vi "Kill Loader.vi"(10 "Log":bool=TRUE, 11 "PIDs":u32[](array[numeric])) -> (0 "error out":errorcluster, 2 "Failed to stop":bool, 3 "Kill Action":T1(ring))   [LabVIEW 2021, in "CIFPluginManager.lvclass"]
uses:
  CIFPluginManager.lvclass
  <vilib>/CIF Foundation/CIF Core/CIFCore/Common/Typedef/Errors.ctl
  typedef/Kill Statemachine.ctl
  <vilib>/CIF Foundation/CIF Core/CIFUtilities/CIFLogs/Typedef/Message Type.ctl
  <vilib>/CIF Foundation/CIF Utilities/Errors/Append Error Location.vi
  <vilib>/CIF Foundation/CIF Core/CIFUtilities/CIFLogs/CIFLogs.lvlib
  <vilib>/CIF Foundation/CIF Core/CIFCore/Common/CIFCoreCommon.lvlib
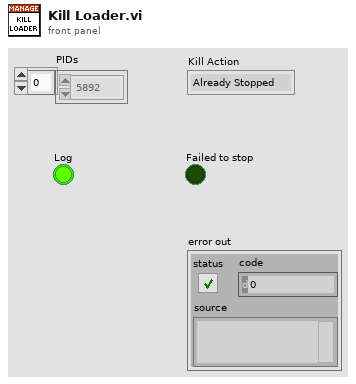
[diagram p1: front panel]
types:
  T1 = enum16{"Already Stopped", "SigInt", "SigTerm", "SigKill"}
  T2 = typedef "CIFCoreCommon.lvlib/Errors.ctl" = enum16{"Invalid Clock ID", "Long Sleep", "gRPC Server Not Found", "Config Parse", "Timestamp Wrap", "Delayed Execution", "Duplicate Channel", "Missing Channel", "Incorrect Type", "Flatten Error", "Unflatten Data", "Unique Name", "Plugin Not Found", "Plugin Type Not Found", "Plugin Version Not Found", "Manager Not Found", "Numerical Issue", "Time Jump", "Clock ID Match", "Channel Length", "Plugin Connection", "gRPC Server Connection", "PPL Name Match", "Build", "Config Log Parse", "Plugin Load", "UI Subpanel Load", "Python Name", "Invalid Name", "Unable to Change Ch Buffer", "Failed Kill", "Failed SysExec", "Function Not Implemented", "Load Timeout"}
  T3 = typedef "CIFPluginManager.lvclass/Kill Statemachine.ctl" = enum16{"Check for Running", "Sleep", "SigInt", "SigTerm", "SigKill"}
  T4 = typedef "CIFLogs.lvlib/Message Type.ctl" = enum16{"Error", "Information", "Print Terminal", "Configuration"}
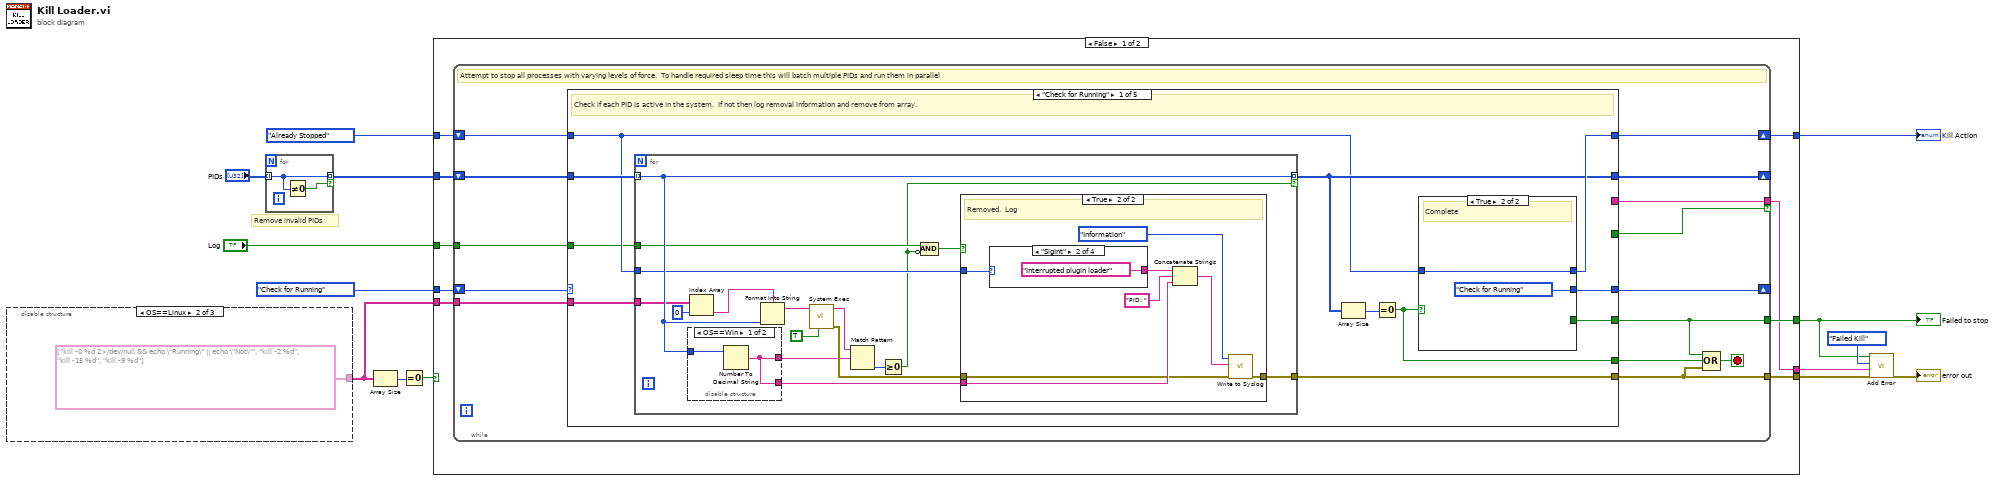
[diagram p0: block diagram]
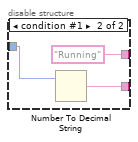
[diagram p2: hidden frame]
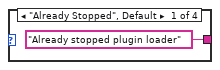
[diagram p4: hidden frame]
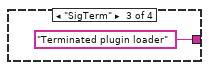
[diagram p5: hidden frame]
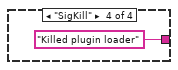
[diagram p6: hidden frame]
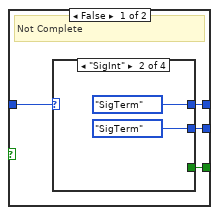
[diagram p7: hidden frame]
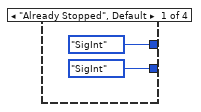
[diagram p8: hidden frame]
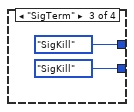
[diagram p9: hidden frame]
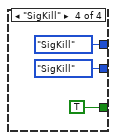
[diagram p10: hidden frame]
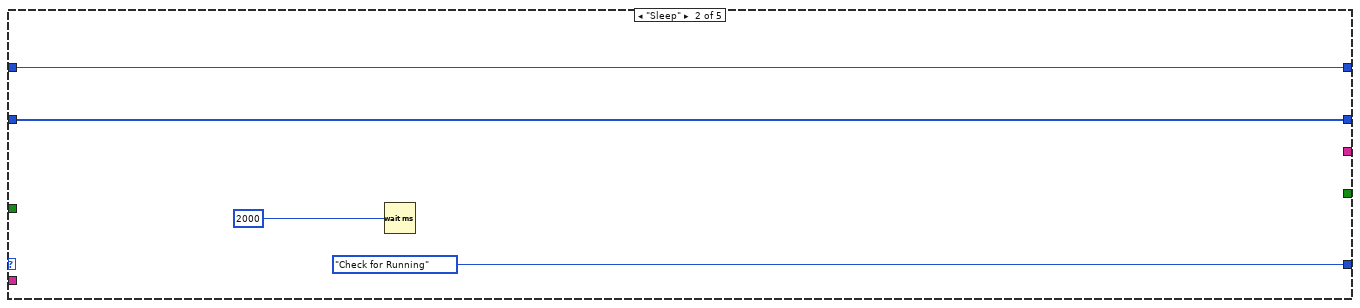
[diagram p11: hidden frame]
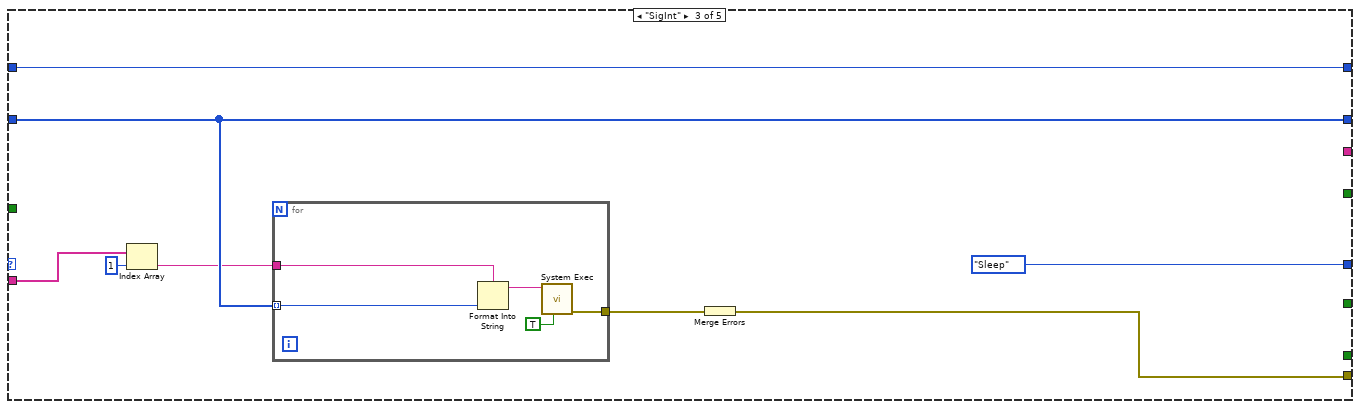
[diagram p12: hidden frame]
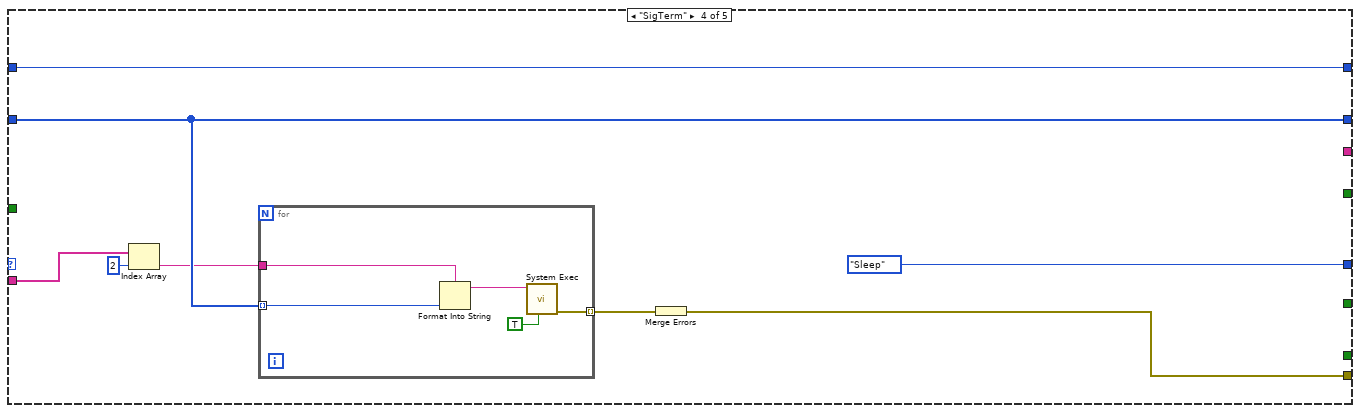
[diagram p13: hidden frame]
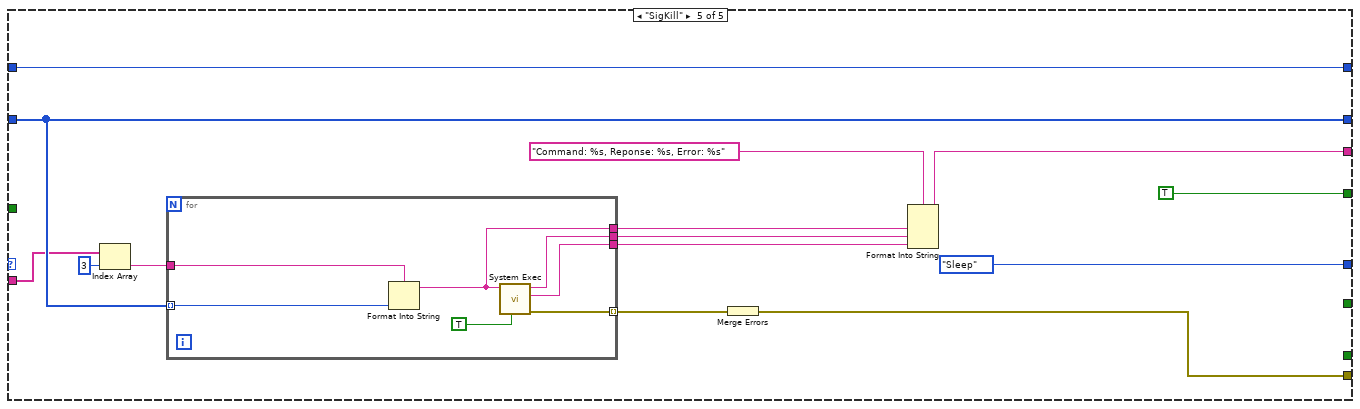
[diagram p14: hidden frame]
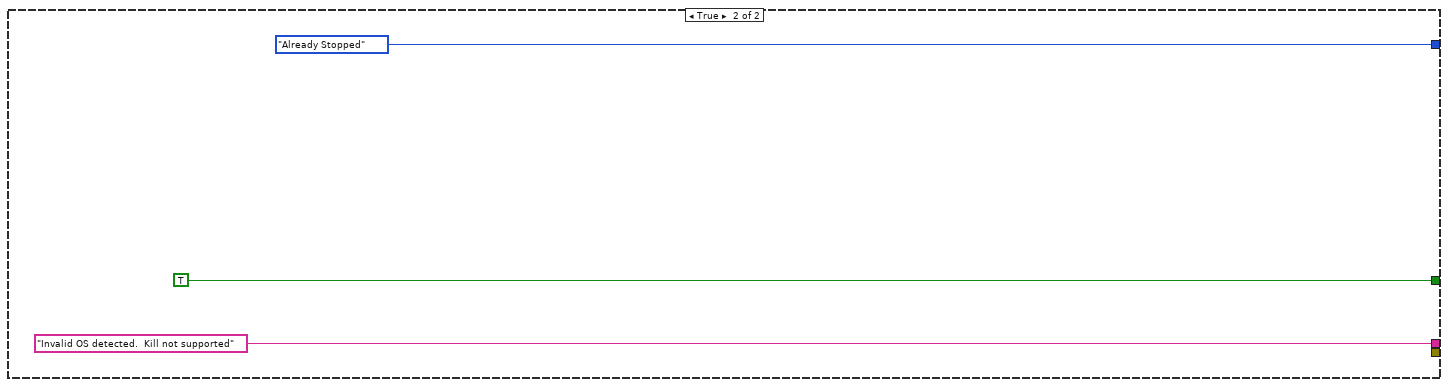
[diagram p15: hidden frame]
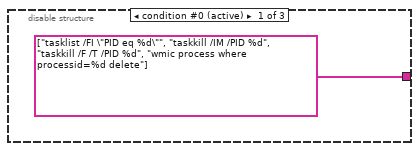
[diagram p16: hidden frame]
diagram:
  # "Remove invalid PIDs"
  n1 = disable-structure shown="OS==Linux" {
    disable-tunnel: [string[] ["tasklist /FI \"PID eq %d\"", "taskkill /IM /PID %d", "taskkill /F /T /PID %d", "wmic process where processid=%d delete"] string[] ["kill -0 %d 2>/dev/null && echo \"Running\" || echo \"Not\"", "kill -2 %d", "kill -15 %d", "kill -9 %d"] _] -> w3
    frame condition #0 (active) {
    }
    frame condition #1 {
    }
    frame condition #2 {
    }
  }
  n2 = for {
    tunnel: "PIDs" -> [w18] mode=indexing
    tunnel: [w18] -> w10 mode=indexing if=w17
    n3 = Not Equal To 0?(x=w18) -> (x != 0?=w17:bool)
  }
  n4 = Array Size(array=w3) -> (size(s)=w4:i32)
  n5 = Equal To 0?(x=w4) -> (x = 0?=w1:bool)
  n6 = case shown="False" w1 {
    tunnel: Kill_Statemachine."Check for Running" ("Kill Statemachine") -> [w27 _]
    tunnel: T1."Already Stopped" ("Kill Result") -> [w26 _]
    tunnel: [w25 T1."Already Stopped" ("Kill Result")] -> w12
    tunnel: w10 -> [w24 _]
    tunnel: [w23 _] -> w8
    tunnel: [w22 TRUE] -> w2
    tunnel: [w21 "Invalid OS detected.  Kill not supported"] -> w6
    tunnel: "Log" -> [w20 _]
    tunnel: w3 -> [w19 _]
    frame False {
      n7 = while {
        shift-right: [w39] -> _
        shift-left: w27 -> [w41]
        shift-right: [w38] -> w25
        shift-left: w26 -> [w40]
        tunnel: [w31] -> w22
        tunnel: [w36] -> w21 if=w35
        tunnel: [w34] -> w23
        shift-right: [w32] -> _
        shift-left: w24 -> [w33]
        tunnel: w20 -> [w29]
        tunnel: w19 -> [w28]
        stop <- w37 stop-if-true
        # "Attempt to stop all processes with varying levels of force.  To handle required sleep time this will batch multiple PIDs and run them in parallel"
        n8 = case shown="\"Check for Running\"" w41 {
          tunnel: [w45 _ _ _ _] -> w30
          tunnel: w40 -> [w44 w105 w113 w126 w145]
          tunnel: [w52 w105 w113 w126 w145] -> w38
          tunnel: [w51 Kill_Statemachine."Check for Running" ("Kill Statemachine") Kill_Statemachine."Sleep" ("Kill Statemachine") Kill_Statemachine."Sleep" ("Kill Statemachine") Kill_Statemachine."Sleep" ("Kill Statemachine")] -> w39
          tunnel: [w50 _ _ _ _] -> w31
          tunnel: [_ _ _ _ w139] -> w36
          tunnel: [_ _ _ _ TRUE] -> w35
          tunnel: [w49 _ w109 w123 w136] -> w34
          tunnel: w33 -> [w48 w102 w111 w122 w135]
          tunnel: [w46 w102 w111 w122 w135] -> w32
          tunnel: w29 -> [w43 _ _ _ _]
          tunnel: w28 -> [w42 _ w107 w119 w132]
          frame "Check for Running" {
            # "Check if each PID is active in the system.  If not then log removal information and remove from array."
            n9 = for {
              tunnel: [w61] -> w49
              tunnel: w48 -> [w64] mode=indexing
              tunnel: [w64] -> w46 mode=indexing if=w59
              tunnel: w44 -> [w63]
              tunnel: w43 -> [w60]
              tunnel: w42 -> [w57]
              n10 = disable-structure shown="OS==Win" {
                disable-tunnel: w64 -> [w70 w72]
                disable-tunnel: [w69 "Running"] -> w54
                disable-tunnel: [w69 w71] -> w53
                frame condition #0 (active) {
                  n11 = Number To Decimal String(number=w70) -> (decimal integer string=w69:string)  [unwired: 1 in]
                }
                frame condition #1 {
                  n12 = Number To Decimal String(number=w72) -> (decimal integer string=w71:string)  [unwired: 1 in]
                }
              }
              n13 = Index Array(array=w57, index=0) -> (element=w56:string)
              n14 = Format Into String(format string=w56, w64) -> (resulting string=w68:string)  [unwired: 2 in, 1 out]
              n15 = call <vilib>:"System Exec.vi"("run minimized? (F)"=TRUE, "command line"=w68) -> ("error out"=w62:errorcluster, "standard output"=w66:string)  [unwired: 6 in, 2 out]
              n16 = Match Pattern(string=w66, regular expression=w54) -> (offset past match=w65:i32)  [unwired: 1 in, 3 out]
              n17 = Greater Or Equal To 0?(x=w65) -> (x >= 0?=w59:bool)
              n18 = Compound Arithmetic op=AND(w60, invert w59) -> (w58:bool)
              n19 = case shown="True" w58 {
                tunnel: w53 -> [_ w81]
                tunnel: w63 -> [_ w79]
                tunnel: w62 -> [w74 w77]
                tunnel: [w74 w76] -> w61
                frame False {
                  # "Not Removed"
                }
                frame True {
                  # "Removed.  Log"
                  n20 = case shown="\"SigInt\"" w79 {
                    tunnel: ["Already stopped plugin loader" ("message") "Interrupted plugin loader" ("message") "Terminated plugin loader" ("message") "Killed plugin loader" ("message")] -> w82
                    frame "Already Stopped", Default {
                    }
                    frame "SigInt" {
                    }
                    frame "SigTerm" {
                    }
                    frame "SigKill" {
                    }
                  }
                  n21 = Concatenate Strings(w82, "PID: " ("message"), w81) -> (w75:string)
                  n22 = call <vilib>:"Write to Syslog.vi"("error in (no error)"=w77, "message"=w75, "CIF Message Type"=Message_Type."Information") -> ("error out"=w76:errorcluster)  [unwired: 8 in]
                }
              }
            }
            n23 = Array Size(array=w46) -> (size(s)=w47:i32)
            n24 = Equal To 0?(x=w47) -> (x = 0?=w45:bool)
            n25 = case shown="True" w45 {
              tunnel: w44 -> [w90 w101]
              tunnel: [w88 w101] -> w52
              tunnel: [w89 Kill_Statemachine."Check for Running" ("Kill Statemachine")] -> w51
              tunnel: [w87 _] -> w50
              frame False {
                # "Not Complete"
                n26 = case shown="\"SigInt\"" w90 {
                  tunnel: [Kill_Statemachine."SigInt" ("Kill Statemachine") Kill_Statemachine."SigTerm" ("Kill Statemachine") Kill_Statemachine."SigKill" ("Kill Statemachine") Kill_Statemachine."SigKill" ("Kill Statemachine")] -> w89
                  tunnel: [T1."SigInt" ("Kill Result") T1."SigTerm" ("Kill Result") T1."SigKill" ("Kill Result") T1."SigKill" ("Kill Result")] -> w88
                  tunnel: [_ _ _ TRUE] -> w87
                  frame "Already Stopped", Default {
                  }
                  frame "SigInt" {
                  }
                  frame "SigTerm" {
                  }
                  frame "SigKill" {
                  }
                }
              }
              frame True {
                # "Complete"
              }
            }
          }
          frame "Sleep" {
            n27 = Wait (ms)(milliseconds to wait=u32 2000) -> ()  [unwired: 1 out]
          }
          frame "SigInt" {
            n28 = Index Array(array=w107, index=1) -> (element=w106:string)
            n29 = for {
              tunnel: w111 -> [w116] mode=indexing
              tunnel: [w115] -> w110
              tunnel: w106 -> [w114]
              n30 = Format Into String(format string=w114, w116) -> (resulting string=w118:string)  [unwired: 2 in, 1 out]
              n31 = call <vilib>:"System Exec.vi"("run minimized? (F)"=TRUE, "command line"=w118) -> ("error out"=w115:errorcluster)  [unwired: 6 in, 3 out]
            }
            n32 = Merge Errors(w110) -> (w109:errorcluster)
          }
          frame "SigTerm" {
            n33 = Index Array(array=w119, index=2) -> (element=w120:string)
            n34 = for {
              tunnel: w122 -> [w129] mode=indexing
              tunnel: [w128] -> w124 mode=indexing
              tunnel: w120 -> [w127]
              n35 = Format Into String(format string=w127, w129) -> (resulting string=w131:string)  [unwired: 2 in, 1 out]
              n36 = call <vilib>:"System Exec.vi"("run minimized? (F)"=TRUE, "command line"=w131) -> ("error out"=w128:errorcluster)  [unwired: 6 in, 3 out]
            }
            n37 = Merge Errors(w124) -> (w123:errorcluster)
          }
          frame "SigKill" {
            n38 = Index Array(array=w132, index=3) -> (element=w133:string)
            n39 = for {
              tunnel: w135 -> [w151] mode=indexing
              tunnel: [w150] -> w142
              tunnel: [w149] -> w141
              tunnel: [w148] -> w140
              tunnel: [w147] -> w137 mode=indexing
              tunnel: w133 -> [w146]
              n40 = Format Into String(format string=w146, w151) -> (resulting string=w150:string)  [unwired: 2 in, 1 out]
              n41 = call <vilib>:"System Exec.vi"("run minimized? (F)"=TRUE, "command line"=w150) -> ("error out"=w147:errorcluster, "standard error"=w148:string, "standard output"=w149:string)  [unwired: 6 in, 1 out]
            }
            n42 = Merge Errors(w137) -> (w136:errorcluster)
            n43 = Format Into String(format string="Command: %s, Reponse: %s, Error: %s" ("initial string"), w142, w141, w140) -> (resulting string=w139:string)  [unwired: 2 in, 1 out]
          }
        }
        n44 = Compound Arithmetic op=OR(w31, w30, w34) -> (w37:bool)
      }
    }
    frame True {
    }
  }
  "Failed to stop" <- w2
  "Kill Action" <- w12
  n45 = call <vilib>:"Add Error.vi"("error in (no error)"=w8, "String to Append"=w6, "Error"=Errors."Failed Kill", "Insert Error"=w2) -> ("error out"=→"error out":errorcluster)  [unwired: 7 in]
